vi "GT_LmtsOff.vi"(3 "limitType":i16(ring) items=["MC_LIMIT_POSITIVE", "MC_LIMIT_NEGATIVE", "BOTH"], 4 "axis":i16, 5 "rtn_In":cluster{"rtn":i16, "Func":string}) -> (1 "axis out":i16, 2 "rtn_Out":cluster{"rtn":i16, "Func":string})   [LabVIEW 2014]
uses:
  VC6/gts.dll
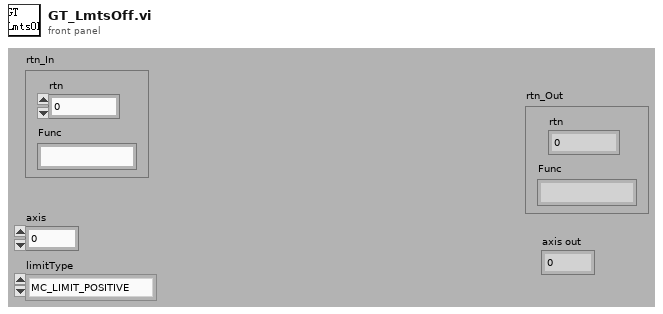
[diagram p1: front panel]
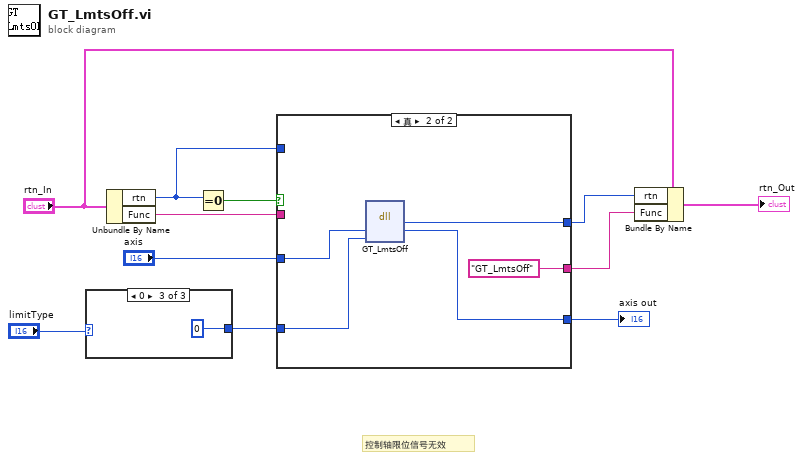
[diagram p0: block diagram]
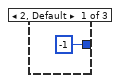
[diagram p2: hidden frame]
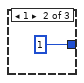
[diagram p3: hidden frame]
diagram:
  # "控制轴限位信号无效"
  n1 = case shown="0" "limitType" {
    tunnel: [i16 -1 ("limitType") i16 1 ("limitType") i16 0 ("limitType")] -> w4
    frame 2, Default {
    }
    frame 1 {
    }
    frame 0 {
    }
  }
  n2 = Unbundle By Name("rtn_In") -> ("rtn"=w3:i16, "Func"=w2:string)
  n3 = Equal To 0?(x=w3) -> (x = 0?=w11:bool)
  n4 = case shown="真" w11 {
    tunnel: "axis" -> [w15 w22]
    tunnel: [w17 w21] -> w7
    tunnel: [w16 "GT_LmtsOff" ("Func")] -> w6
    tunnel: w4 -> [_ w19]
    tunnel: w3 -> [w17 _]
    tunnel: w2 -> [w16 _]
    tunnel: [w15 w18] -> w1
    frame False {
    }
    frame True {
      n5 = dll-call lib="PTH2Fabs DNewGTS AC-800LWin7版源程序-20170926gts85VC6gts.dll" fn="GT_LmtsOff"("axis"=w22, "limitType"=w19) -> ("rtn"=w21:i16, "axis"=w18:i16)  [unwired: 4 in, 2 out]
    }
  }
  "axis out" <- w1
  n6 = Bundle By Name(cluster="rtn_In", "rtn"=w7, "Func"=w6) -> (→"rtn_Out":cluster{"rtn":i16, "Func":string})
